vi "GOLPI Rebuild Start and Stop Commands.vi"(7 "processing setup":T1={"mode"=enum."Raw", "call after avgs?"=FALSE, "calculate?"=FALSE, "raw mode"={"command"="", "result mode"=enum."Display console output (only Octave)", "res variable"=""}, "QWTB"={"QWTB path"=path "", "alg filter path"="", "alg ids"=[], "alg parameters"=[], "parsed parameters"=[], "selected alg id"="", "selected unc mode"=enum."None", "qwtb mcc"=100, "qwtb timeout"=90, "qwtb covg"=95.0, "qwtb ofs"=0, "qwtb lim data"=0, "multicore"={"jobs folder"=path "", "cores"=0, "max jobs"=0, "mode"=enum."Singlecore"}, "unc once?"=FALSE}}, 8 "error in":errorcluster, 11 "golpi session in":T10={"GOLPI ref"={"pipe handle"={"lv_proc.dll file path"=path "", "process instance handle"=[], "debug mode"=FALSE, "debug data"=[]}, "fast read timeout [ms]"=500, "fast read settle time [ms]"=10, "fast read to multiple [ms]"=1, "max elements per input line"=100, "slow read timeout [ms]"=5000, "stdin double format specifier"="%_16e", "max elements per stdout output column"=100, "console mode bitstream"=FALSE, "bitstream first read timeout [ms]"=1000, "bitstream read timeout [ms]"=50, "struct transfer possible"=FALSE, "matlab mode"=FALSE}, "idn str"="", "octave path"=path "C:/Octave364/Octave3.6.4_gcc4.6.2/bin", "work path"=path "C:/Octave364/Octave3.6.4_gcc4.6.2/bin", "start timeout [ms]"=15000, "clr cache"=FALSE, "console"=FALSE, "binary"=FALSE, "semaphore"=refnum, "initial command"="", "exit command"="", "matlab"=FALSE}) -> (0 "error out":errorcluster, 3 "golpi session out":T10={"GOLPI ref"={"pipe handle"={"lv_proc.dll file path"=path "", "process instance handle"=[], "debug mode"=FALSE, "debug data"=[]}, "fast read timeout [ms]"=500, "fast read settle time [ms]"=10, "fast read to multiple [ms]"=1, "max elements per input line"=100, "slow read timeout [ms]"=5000, "stdin double format specifier"="%_16e", "max elements per stdout output column"=100, "console mode bitstream"=FALSE, "bitstream first read timeout [ms]"=1000, "bitstream read timeout [ms]"=50, "struct transfer possible"=FALSE, "matlab mode"=FALSE}, "idn str"="", "octave path"=path "C:/Octave364/Octave3.6.4_gcc4.6.2/bin", "work path"=path "C:/Octave364/Octave3.6.4_gcc4.6.2/bin", "start timeout [ms]"=15000, "clr cache"=FALSE, "console"=FALSE, "binary"=FALSE, "semaphore"=refnum, "initial command"="", "exit command"="", "matlab"=FALSE})   [LabVIEW 2018]
doc: "This will rebuild initial command sequence that is issued when Octave/Matlab starts or before Octave/Matlab ends."
uses:
  golpi_session.ctl
  GOLPI Library.lvlibp/Public/GOLPI reference Type Def.ctl
  GOLPI Library.lvlibp/LV Process source distribution/Pipe Handle.ctl
  measure/processing/Meas Process Config.ctl
  measure/processing/Meas Process Mode.ctl
  measure/processing/Meas Process Raw Config.ctl
  measure/processing/Meas Process Raw Result Mode.ctl
  measure/processing/QWTB/Meas Proc QWTB Setup.ctl
  measure/processing/QWTB/Meas Proc QWTB Algorithm Parameter Data.ctl
  measure/processing/QWTB/Meas Proc QWTB Uncertainty Mode.ctl
  measure/processing/QWTB/Meas Proc QWTB Multicore Setup.ctl
  measure/processing/QWTB/Meas Proc QWTB Multicore Type.ctl
  GOLPI Library.lvlibp/LV Process source distribution/LV Process library.lvlib
  GOLPI Library.lvlibp
  GOLPI Multi Process.lvlib
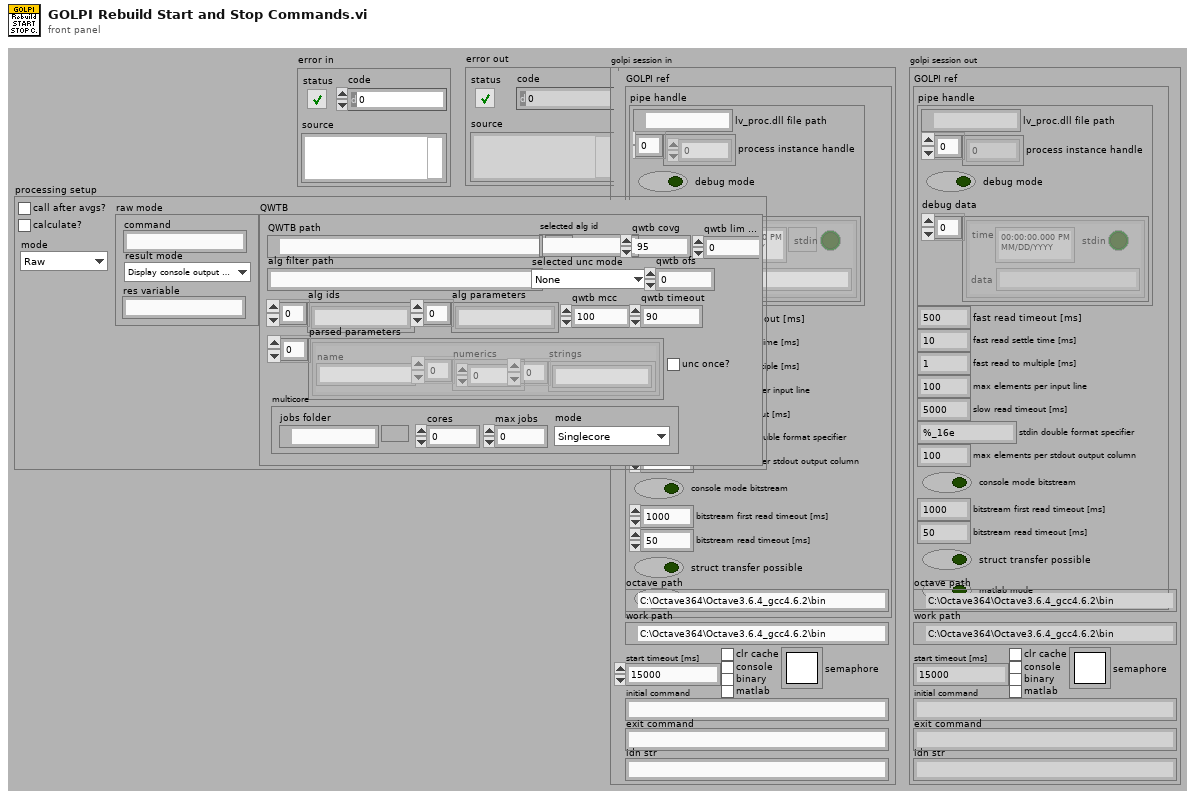
[diagram p1: front panel]
types:
  T1 = typedef "Meas Process Config.ctl" = cluster{"mode":T2, "call after avgs?":bool, "calculate?":bool, "raw mode":T3, "QWTB":T5}
  T2 = typedef "Meas Process Mode.ctl" = enum16{"Raw", "QWTB"}
  T3 = typedef "Meas Process Raw Config.ctl" = cluster{"command":string, "result mode":T4, "res variable":string}
  T4 = typedef "Meas Process Raw Result Mode.ctl" = enum16{"Display console output (only Octave)", "Display string variable", "Display result file %respath%"}
  T5 = typedef "Meas Proc QWTB Setup.ctl" = cluster{"QWTB path":path, "alg filter path":string, "alg ids":string[], "alg parameters":string[], "parsed parameters":T6[], "selected alg id":string, "selected unc mode":T7, "qwtb mcc":i32, "qwtb timeout":i32, "qwtb covg":dbl, "qwtb ofs":i64, "qwtb lim data":i64, "multicore":T8, "unc once?":bool}
  T6 = typedef "Meas Proc QWTB Algorithm Parameter Data.ctl" = cluster{"name":string, "numerics":dbl[], "strings":string[]}
  T7 = typedef "Meas Proc QWTB Uncertainty Mode.ctl" = enum16{"None", "GUF", "Monte Carlo"}
  T8 = typedef "Meas Proc QWTB Multicore Setup.ctl" = cluster{"jobs folder":path, "cores":i32, "max jobs":i32, "mode":T9}
  T9 = typedef "Meas Proc QWTB Multicore Type.ctl" = enum16{"Singlecore", "Multicore", "Multistation"}
  T10 = typedef "GOLPI Multi Process.lvlib/golpi_session.ctl" = cluster{"GOLPI ref":T11, "idn str":string, "octave path":path, "work path":path, "start timeout [ms]":u32, "clr cache":bool, "console":bool, "binary":bool, "semaphore":T13, "initial command":string, "exit command":string, "matlab":bool}
  T11 = typedef "GOLPI Library.lvlibp/GOLPI reference Type Def.ctl" = cluster{"pipe handle":T12, "fast read timeout [ms]":u32, "fast read settle time [ms]":u32, "fast read to multiple [ms]":u32, "max elements per input line":u32, "slow read timeout [ms]":u32, "stdin double format specifier":string, "max elements per stdout output column":u32, "console mode bitstream":bool, "bitstream first read timeout [ms]":u32, "bitstream read timeout [ms]":u32, "struct transfer possible":bool, "matlab mode":bool}
  T12 = typedef "GOLPI Library.lvlibp/LV Process library.lvlib/Pipe Handle.ctl" = cluster{"lv_proc.dll file path":path, "process instance handle":u32[], "debug mode":bool, "debug data":cluster{"time":timestamp, "stdin":bool, "data":string}[]}
  T13 = typedef "Semaphore RefNum" = refnum<k1>
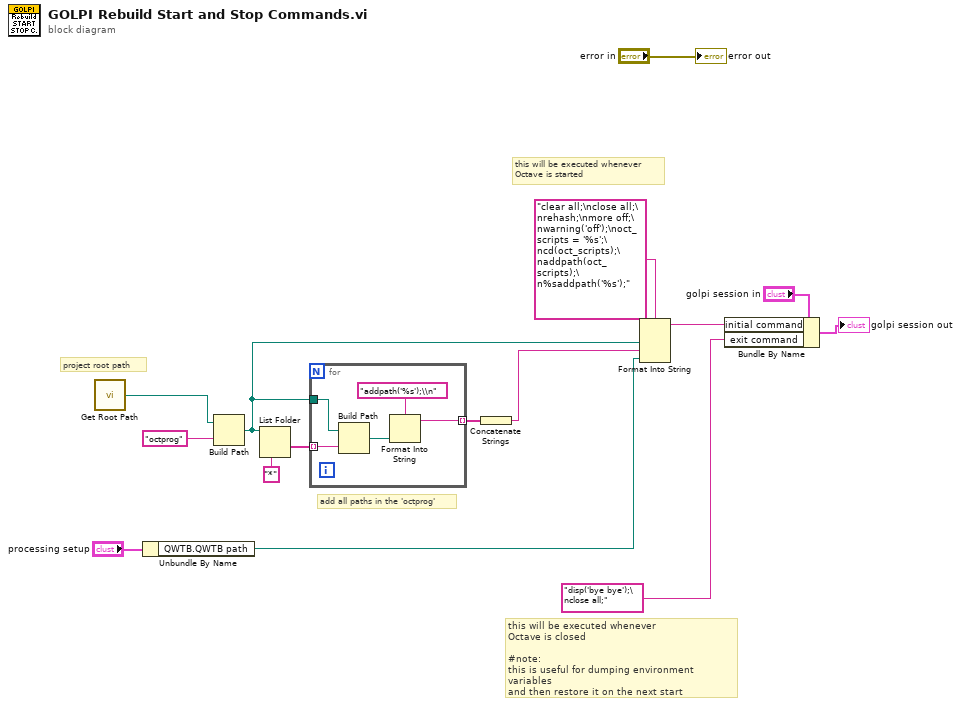
[diagram p0: block diagram]
diagram:
  # "add all paths in the 'octprog'"
  # "project root path"
  # "this will be executed whenever\nOctave is closed\n\n#note: \nthis is useful for dumping environment variables\nand then restore it on the next start"
  # "this will be executed whenever\nOctave is started"
  n1 = call "Get Root Path.vi"() -> ("root path"=w1:path)
  n2 = Unbundle By Name("processing setup") -> ("QWTB.QWTB path"=w3:path)
  n3 = Build Path(base path=w1, name or relative path="octprog") -> (appended path=w2:path)
  n4 = List Folder(path=w2, pattern="*") -> (folder names=w7:string[])  [unwired: 2 in, 3 out]
  n5 = for {
    tunnel: w7 -> [w20] mode=indexing
    tunnel: w2 -> [w19]
    tunnel: [w16] -> w6 mode=indexing
    n6 = Build Path(base path=w19, name or relative path=w20) -> (appended path=w18:path)
    n7 = Format Into String(format string="addpath('%s');\\n", w18) -> (resulting string=w16:string)  [unwired: 2 in, 1 out]
  }
  n8 = Concatenate Strings(w6) -> (w5:string)
  n9 = Format Into String(format string="clear all;\nclose all;\nrehash;\nmore off;\nwarning('off');\noct_scripts = '%s';\ncd(oct_scripts);\naddpath(oct_scripts);\n%saddpath('%s');", w2, w5, w3) -> (resulting string=w13:string)  [unwired: 2 in, 1 out]
  n10 = Bundle By Name(cluster="golpi session in", "initial command"=w13, "exit command"="disp('bye bye');\nclose all;" ("format string")) -> (→"golpi session out":T10)
  "error out" <- "error in"
